vi "InitiateRFSAPeer2Peer.vi"(8 "error in (no error)":errorcluster, 11 "vi path":path=path "C:/Users/LocalAdmin/Documents/VST-7902 Aurora/Host/RFSA Peer-to-Peer Host with FFT.vi") -> (0 "error out":errorcluster, 3 "vi reference":refnum<vi>)   [LabVIEW 2019]
panel:
  out "Boolean":bool=TRUE
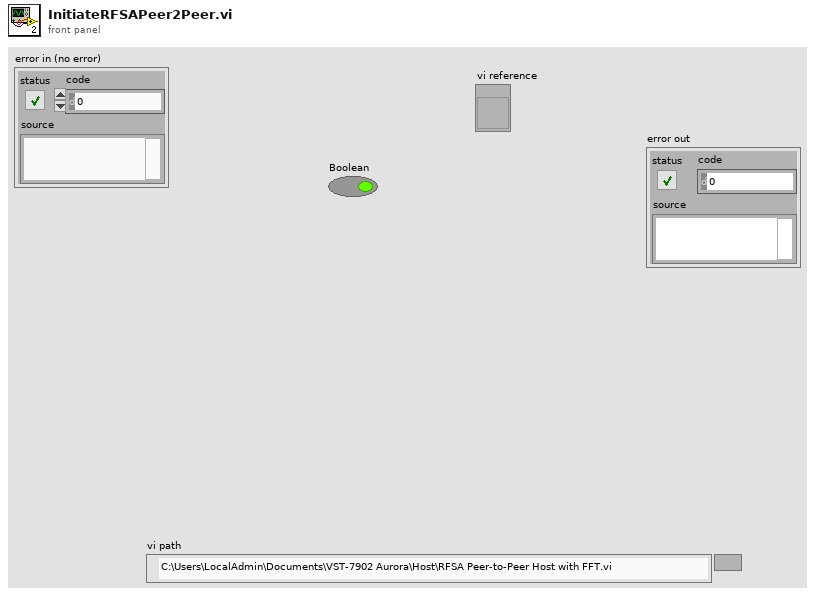
[diagram p1: front panel]
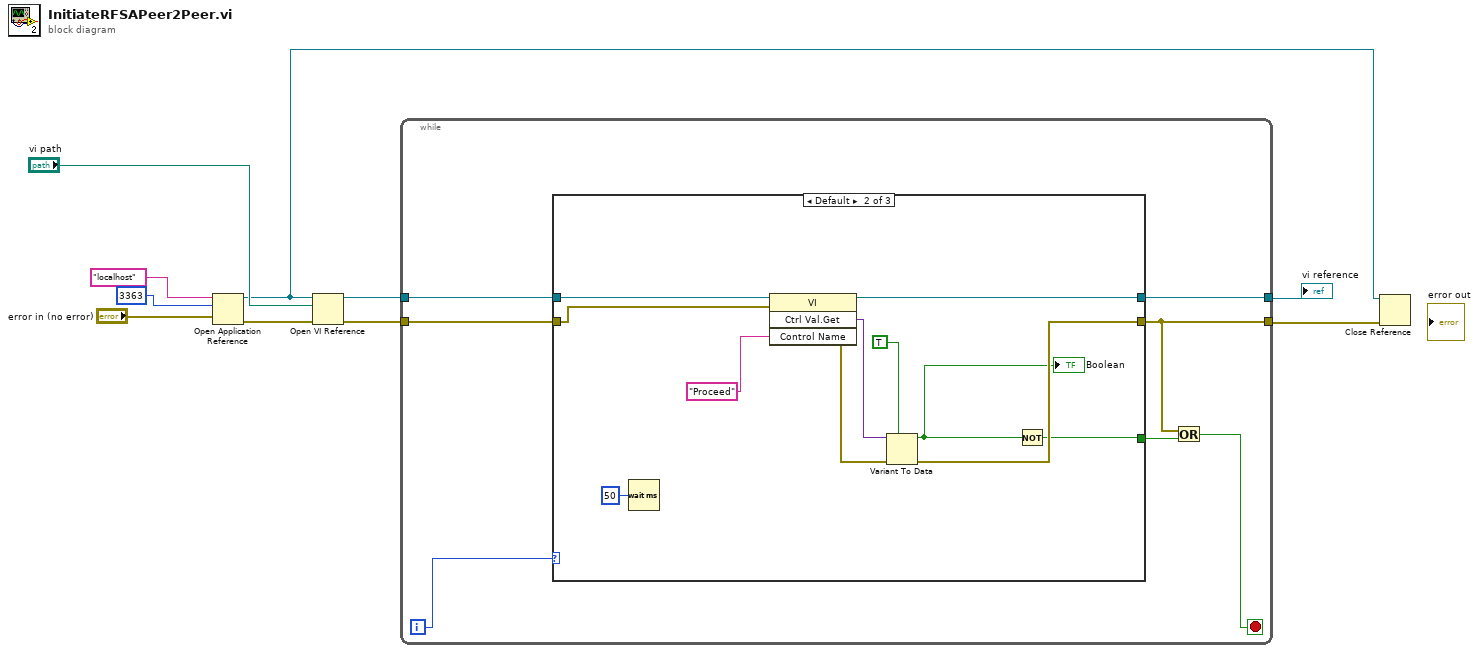
[diagram p0: block diagram]
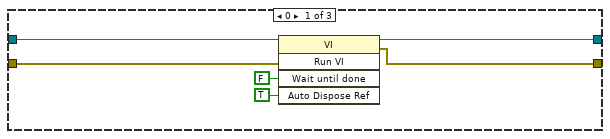
[diagram p2: hidden frame]
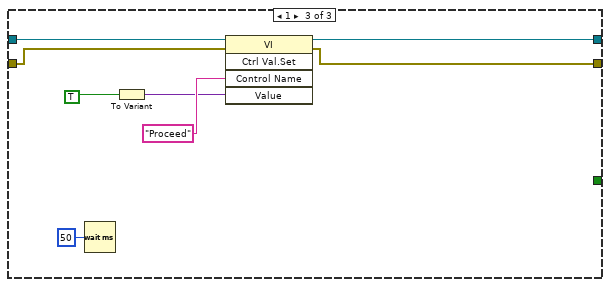
[diagram p3: hidden frame]
diagram:
  n1 = Open Application Reference(8:"error in (no error)", 10:u16 3363 ("port number or service name (3363)"), 11:"localhost" ("machine name (\"\":  open local reference)")) -> (0:w9:errorcluster, 3:w2:refnum<vi>)  [unwired: 1 in]
  n2 = Open VI Reference(application reference (local)=w2, vi path="vi path", error in (no error)=w9) -> (vi reference=w6:refnum<vi>, error out=w5:errorcluster)  [unwired: 3 in]
  n3 = while {
    tunnel: w6 -> [w16]
    tunnel: [w15] -> w3
    tunnel: w5 -> [w14]
    tunnel: [w11] -> w1
    i -> [w17]
    stop <- w12 stop-if-true
    n4 = case shown="Default" w17 {
      tunnel: w16 -> [w22 w33 w41]
      tunnel: [w21 w32 w40] -> w15
      tunnel: w14 -> [w20 w29 w38]
      tunnel: [w23 w31 w42] -> w11
      tunnel: [_ w24 _] -> w13
      frame 0 {
        n5 = invoke class="VI" method="Run VI"(reference=w22, error in=w20, "Wait until done"=FALSE ("Wait Until Done"), "Auto Dispose Ref"=TRUE ("Auto Dispose Reference")) -> (reference out=w21:refnum<vi>, error out=w23:errorcluster)  [unwired: 1 in, 3 out]
      }
      frame Default {
        n6 = Wait (ms)(milliseconds to wait=u32 50) -> ()  [unwired: 1 out]
        n7 = invoke class="VI" method="Ctrl Val.Get"(reference=w33, error in=w29, "Control Name"="Proceed") -> (reference out=w32:refnum<vi>, error out=w34:errorcluster, "Get Control Value Variant"=w25:variant)  [unwired: 1 in, 1 out]
        n8 = Variant To Data(error in=w34, type=TRUE ("Boolean"), Variant=w25) -> (data=w27:bool, error out=w31:errorcluster)
        "Boolean" <- w27
        n9 = Not(x=w27) -> (.not. x?=w24:bool)
      }
      frame 1 {
        n10 = Wait (ms)(milliseconds to wait=u32 50) -> ()  [unwired: 1 out]
        n11 = To Variant(anything=TRUE ("Boolean")) -> (Variant=w35:variant)
        n12 = invoke class="VI" method="Ctrl Val.Set"(reference=w41, error in=w38, "Control Name"="Proceed", "Value"=w35) -> (reference out=w40:refnum<vi>, error out=w42:errorcluster)  [unwired: 1 in, 3 out]
      }
    }
    n13 = Or(x=w11, y=w13) -> (x .or. y?=w12:bool)
  }
  "vi reference" <- w3
  n14 = Close Reference(reference=w2, error in (no error)=w1) -> ()  [unwired: 1 out]
